vi "enum-test.vi"() -> ()   [LabVIEW 2016]
uses:
  SubVis/msgpack_config.ctl
  SubVis/cluster_conversion.ctl
  SubVis/enum_conversion.ctl
  MsgPack.lvlib
panel:
  out "string":string
  in  "MsgPack Config":T1={"Cluster Conversion"=enum."to array", "Enum Conversion"=enum."to uint", "Use ArrayType"=FALSE}
  in  "Enum":enum8{"bla", "foo", "bar", "pingpong"}(ring)
  out "Array":u8[](array[numeric]) format="%.0x"
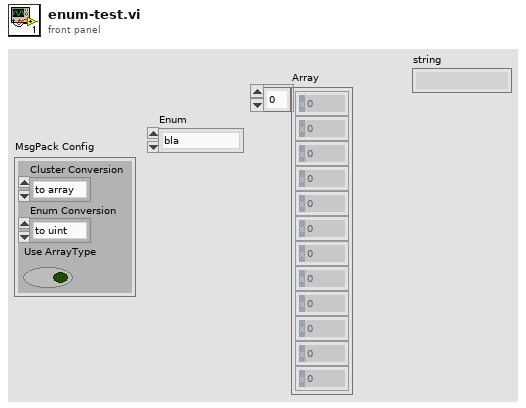
[diagram p1: front panel]
types:
  T1 = typedef "MsgPack.lvlib/msgpack_config.ctl" = cluster{"Cluster Conversion":T2, "Enum Conversion":T3, "Use ArrayType":bool}
  T2 = typedef "MsgPack.lvlib/cluster_conversion.ctl" = enum16{"to map", "to array"}
  T3 = typedef "MsgPack.lvlib/enum_conversion.ctl" = enum16{"to uint", "to string"}
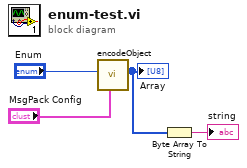
[diagram p0: block diagram]
diagram:
  n1 = call "encodeObject.vi"("MsgPack Config"="MsgPack Config", "Variant"="Enum") -> ("Array"=w2:u8[])  [unwired: 8 in, 1 out]
  "Array" <- w2
  n2 = Byte Array To String(unsigned byte array=w2) -> (string=→"string":string)
